vi "Get Class CSV_File.vi"(8 "error in (no error)":errorcluster caption="entrée d'erreur (pas d'erreur)", 11 "Class Log_File (Default) en entrée":refnum<class "Class Log_File (Default).lvclass">) -> (0 "error out":errorcluster caption="sortie d'erreur", 2 "Library File.lvlib:Class CSV_File.lvclass":refnum<class "Class CSV_File.lvclass">, 3 "Class Log_File (Default) en sortie":refnum<class "Class Log_File (Default).lvclass">)   [LabVIEW 2020, in "Library Instrument & Equipement.lvlib" / "Library Log_File.lvlib" / "Class Log_File (Default).lvclass"]
uses:
  Class Log_File (Default).lvclass
  Read CSV File/CSV_File (Default)/Class CSV_File.lvclass
  Class Log_File (Default).lvclass/Class Log_File (Default).ctl
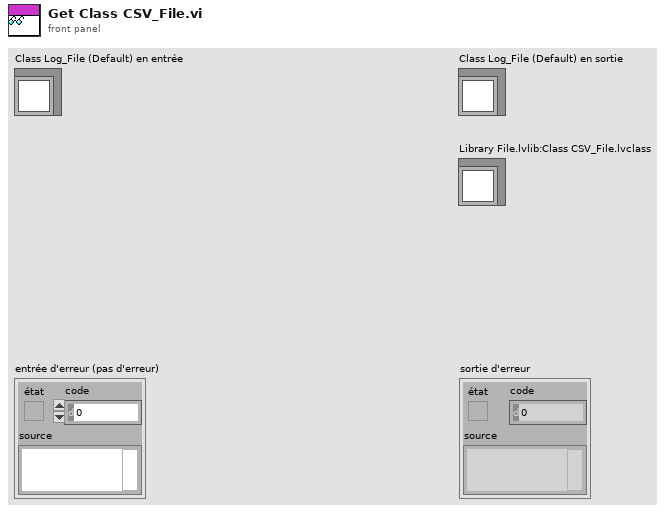
[diagram p1: front panel]
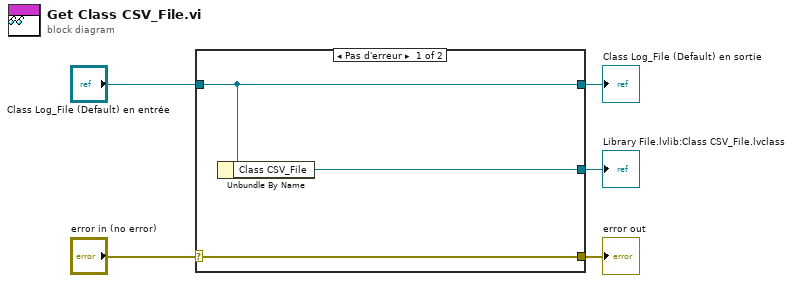
[diagram p0: block diagram]
diagram:
  n1 = case shown="Pas d'erreur" "error in (no error)" {
    selector: "error in (no error)" -> [w8 w9]
    tunnel: [w8 w9] -> w4
    tunnel: [w7 w10] -> w2
    tunnel: "Class Log_File (Default) en entrée" -> [w7 w10]
    tunnel: [w6 _] -> w1
    frame No Error {
      n2 = Unbundle By Name(w7) -> ("Class CSV_File"=w6:refnum<class "Class CSV_File.lvclass">)
    }
    frame Error {
    }
  }
  "error out" <- w4
  "Class Log_File (Default) en sortie" <- w2
  "Library File.lvlib:Class CSV_File.lvclass" <- w1
